vi "dfd_DFXP_Right Shift (vector).vi"(9 "High 64":i64[](array[numeric]), 10 "Low 64":u64[](array[numeric]), 11 "Num":i16) -> (1 "High 64":i64[](array[numeric]), 2 "Low 64":u64[](array[numeric]))   [LabVIEW 2017, in "NI_DigFilter_FXP.lvlib"]
uses:
  <vilib>/addons/Digital Filter Design/NI_DigFilter_FXP.lvlib
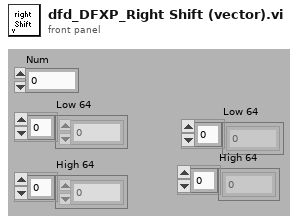
[diagram p1: front panel]
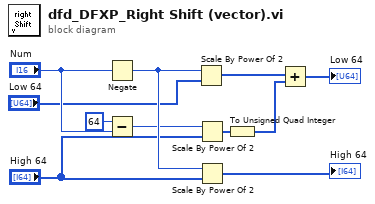
[diagram p0: block diagram]
diagram:
  n1 = Negate(x="Num") -> (-x=w8:i16)
  n2 = Subtract(x=i16 64 ("y"), y="Num") -> (x-y=w7:i16)
  n3 = Scale By Power Of 2(n=w8, x="Low 64") -> (x*2^n=w9:u64[])
  n4 = Scale By Power Of 2(n=w7, x="High 64") -> (x*2^n=w6:i64[])
  n5 = Scale By Power Of 2(n=w8, x="High 64") -> (x*2^n=→"High 64":i64[])
  n6 = To Unsigned Quad Integer(1:w6) -> (0:w5:u64[])
  n7 = Add(x=w9, y=w5) -> (x+y=→"Low 64":u64[])
